vi "Clear LabVIEW Errors.vi"(8 "error in (no error)":errorcluster, 11 "Alarm Handler Actor in":refnum<class "Error Handler Actor.lvclass">) -> (0 "error out":errorcluster, 3 "Alarm Handler Actor out":refnum<class "Error Handler Actor.lvclass">)   [LabVIEW 2026]
uses:
  Error Handler Actor.lvclass
  C:/dev/LabVIEW/LabMelee/Source/Re-use Libraries/Minimal Actor Framework/Actors/Base Actor/Actor/Actor.lvclass
  C:/dev/LabVIEW/LabMelee/Source/Application Specific/Actors/Error Handler/Actor/Error Handler Actor.lvclass
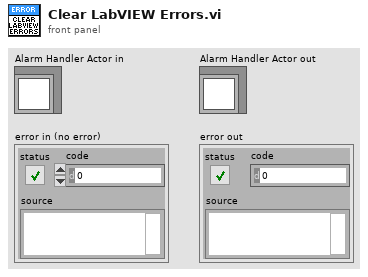
[diagram p1: front panel]
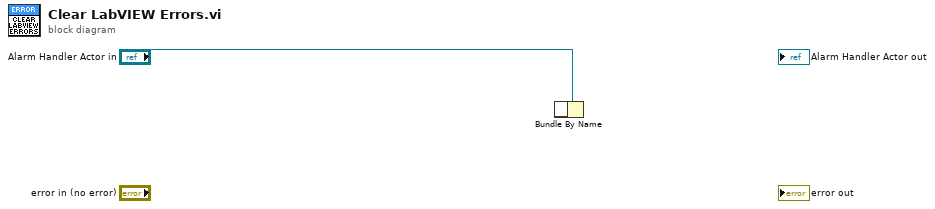
[diagram p0: block diagram]
diagram:
  n1 = Bundle By Name(cluster="Alarm Handler Actor in") -> ()  [unwired: 1 in, 1 out]
